vi "CSMP-Sync Call.vi"(0 "State":string, 1 "Args":string, 2 "Source/target":string, 5 "Error In":errorcluster caption="error in (no error)", 7 "Response Timeout (-2 Using Global Settings)":i32=-2, 8 "Module Name":string) -> (14 "State Out":string, 15 "Args Out":string, 16 "Source/target Out":string, 17 "Pre-State Out":string, 18 "Pre-Args Out":string, 19 "Error":errorcluster)   [LabVIEW 2017, in "Communicable State Machine.lvlib"]
doc: "### CSMP-Sync Call.vi\n\n-- <b>Controls</b> --\n- <b>state</b>:\n- <b>args</b>:\n- <b>source/target</b>:\n- <b>Response Timeout(-2 to use global setting)</b>:\n- <b>Module Name</b>:\n\n-- <b>Indicators</b> --\n- <b>state out</b>:\n- <b>args out</b>:\n- <b>source/target out</b>:\n- <b>Pre-State out</b>:\n- <b>Pre-Args out</b>:\n- <b>error</b>:"
uses:
  Communicable State Machine.lvlib
  Typedef/_Cross CSM State Data.ctl
  Typedef/_CSM_MSG_TYPE.ctl
  Typedef/_Cross CSM State Response.ctl
  Typedef/_CSM_Response Source Message.ctl
  _Shared/CSM - System States.vi
  Priority Queue/Enqueue Element.vi
  AdvanceAPI/CSM - Keywords.vi
  Error/CSM Not Allowed Message.vi
  CSMQ/_CSMOFGV(lvlibp).vi
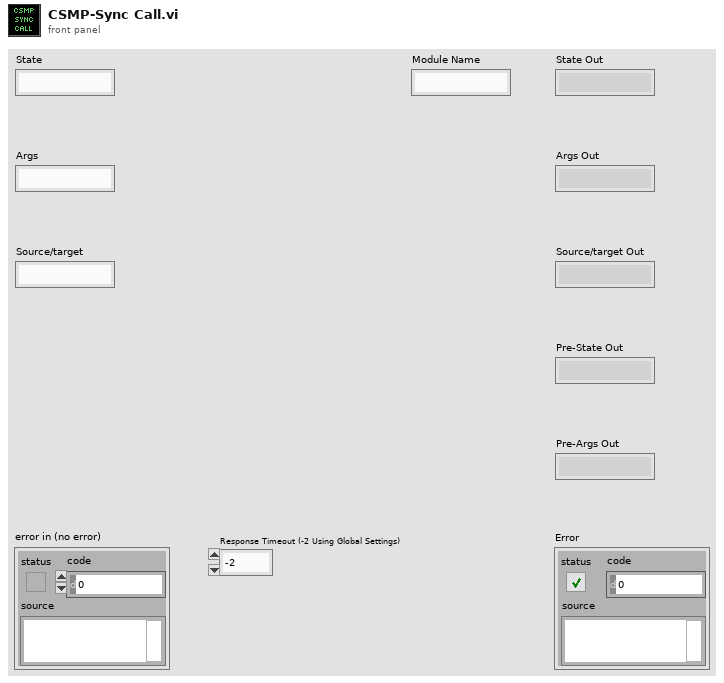
[diagram p1: front panel]
types:
  T1 = typedef "Communicable State Machine.lvlib/_CSMObj.ctl" = cluster{"info":T2, "Refs":T4}
  T2 = typedef "Communicable State Machine.lvlib/_CSMObj-Info.ctl" = cluster{"Module Name":string, "Requested Name":string, "Group Name":string, "Mode":T3, "Allowed Messages":string[]}
  T3 = typedef "Communicable State Machine.lvlib/_CSM_MODE.ctl" = enum16{"Not Exist", "Stand Alone", "CSM", "Worker", "Worker Agent", "Chain Node", "Chain"}
  T4 = typedef "Communicable State Machine.lvlib/_CSMObj-Refs.ctl" = cluster{"WatchDogQ":refnum<queue>, "CSMDataDVR":refnum<data-value>, "Queue":T5, "GroupDataDVR":refnum<data-value>, "TagMap":refnum<data-value>, "ExitEvent":refnum<user-event>, "NewStateEvent":refnum<user-event>, "StatusEvent":refnum<user-event>, "InterruptEvent":refnum<user-event>}
  T5 = typedef "Communicable State Machine.lvlib/Priority Queue.ctl" = cluster{"HPriorityQ":refnum<queue>, "LowPriorityQ":refnum<queue>}
  T6 = typedef "Communicable State Machine.lvlib/_Cross CSM State Response.ctl" = cluster{"error":errorcluster, "Response Data":string, "From Who":string}
  T7 = typedef "Communicable State Machine.lvlib/_CSM_MSG_TYPE.ctl" = enum16{"Sync Message(-@)", "Async Message(->)", "Async without Response(->|)", "Async Response", "Broadcast(-><all>)", "Broadcast(-><status>)", "Broadcast(-><interrupt>)", "Append to JKISM States", "Append to JKISM States(High Priority)", "Broadcast(-><state>)"}
  T8 = typedef "Communicable State Machine.lvlib/_Cross CSM State Data.ctl" = cluster{"Msg Type":T7, "state":string, "args":string, "source":string, "RespQ":refnum<queue>, "Response For Message":T9, "Target":string}
  T9 = typedef "Communicable State Machine.lvlib/_CSM_Response Source Message.ctl" = cluster{"‘State":string, "’Arguments":string, "’Error":errorcluster}
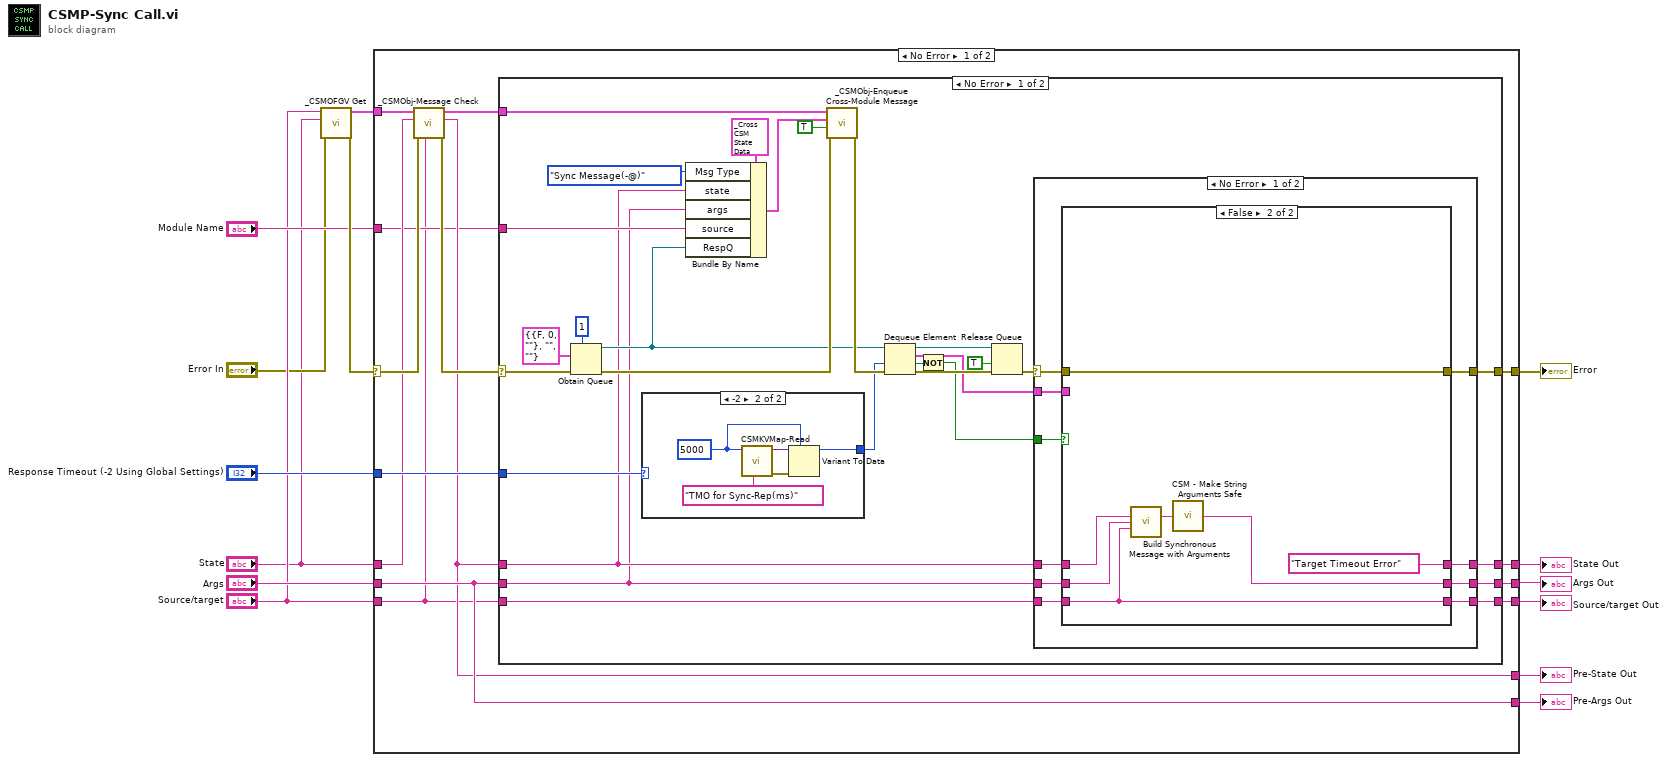
[diagram p0: block diagram]
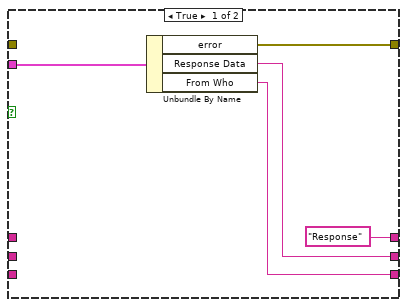
[diagram p2: hidden frame]
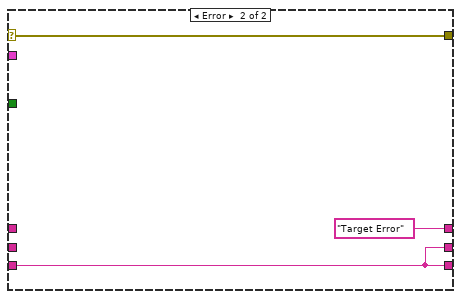
[diagram p3: hidden frame]
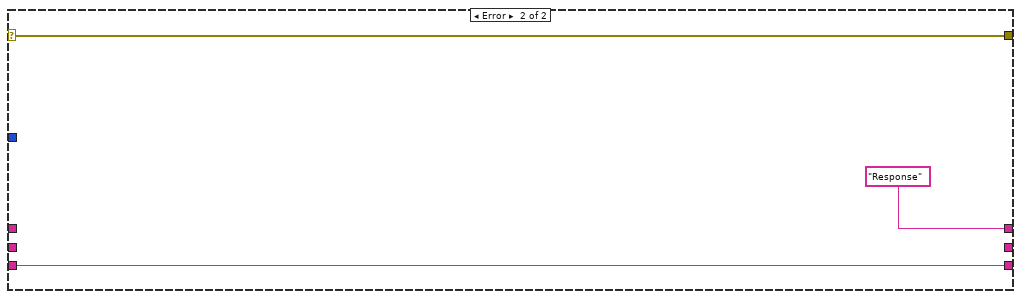
[diagram p5: hidden frame]
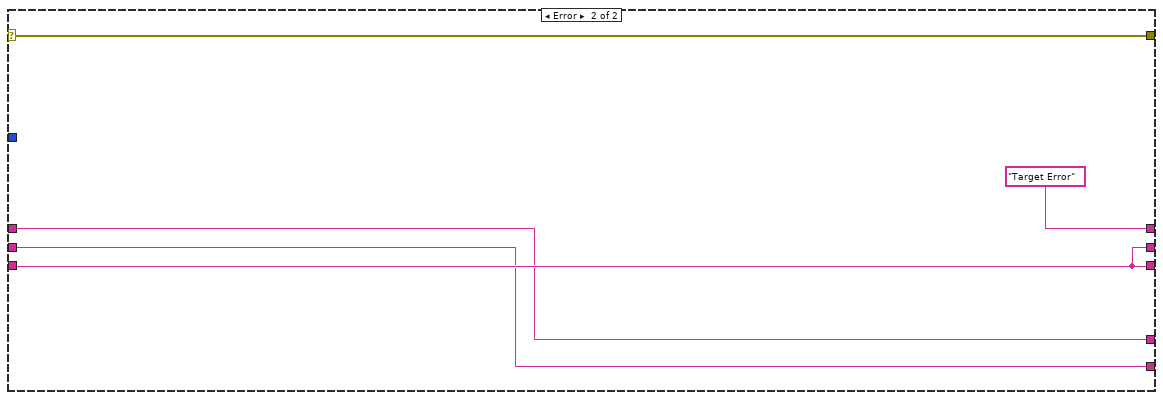
[diagram p6: hidden frame]
diagram:
  n1 = call "_CSMOFGV Get.vi"("Error In"="Error In", "Message"="State", "Name (\"\" to Use UUID) In"="Source/target") -> ("error out"=w13:errorcluster, "CSM-Obj"=w14:T1)  [unwired: 6 in, 1 out]
  n2 = case shown="No Error" w13 {
    selector: w13 -> [w20 w94]
    tunnel: "Response Timeout (-2 Using Global Settings)" -> [w28 _]
    tunnel: w14 -> [w22 _]
    tunnel: [w27 "Target Error" ("before match")] -> w8
    tunnel: [w26 w93] -> w7
    tunnel: "Source/target" -> [w15 w93]
    tunnel: "State" -> [w18 w92]
    tunnel: "Args" -> [w23 w91]
    tunnel: "Module Name" -> [w16 _]
    tunnel: [w23 w91] -> w5
    tunnel: [w25 w94] -> w4
    tunnel: [w17 w92] -> w6
    tunnel: [w24 w93] -> w2
    frame No Error {
      n3 = call "_CSMObj-Message Check.vi"("CSM"=w15, "Error In"=w20, "Message"=w18, "CSMQ In"=w22) -> ("error out"=w19:errorcluster, "Message (Dup)"=w17:string, "CSMQ Out"=w21:T1)  [unwired: 5 in]
      n4 = case shown="No Error" w19 {
        selector: w19 -> [w34 w90]
        tunnel: w28 -> [w32 _]
        tunnel: [w56 "Response" ("f")] -> w27
        tunnel: [w46 _] -> w26
        tunnel: w16 -> [w43 _]
        tunnel: w15 -> [w42 w88]
        tunnel: [w38 w90] -> w25
        tunnel: [w37 w88] -> w24
        tunnel: w23 -> [w29 _]
        tunnel: w21 -> [w35 _]
        tunnel: w17 -> [w30 _]
        frame No Error {
          n5 = Obtain Queue(max queue size (-1, unlimited)=1, element data type=T6 {"error"={"status"=FALSE, "code"=0, "source"=""}, "Response Data"="", "From Who"=""} ("Cross JKI State Machine Response"), error in (no error)=w34) -> (queue out=w45:refnum<queue>, error out=w48:errorcluster)  [unwired: 2 in, 1 out]
          n6 = case shown="-2" w32 {
            selector: w32 -> [w82 _]
            tunnel: [w82 w83] -> w31
            frame 0, Default {
            }
            frame -2 {
              w84 = 5000 ("max queue size (-1, unlimited)")
              n7 = call "CSMKVMap-Read.vi"("name"="TMO for Sync-Rep(ms)", "default value (empty variant)"=w84) -> ("Error out"=w87:errorcluster, "value"=w86:variant)  [unwired: 6 in]
              n8 = Variant To Data(error in=w87, type=w84, Variant=w86) -> (data=w83:i32)  [unwired: 1 out]
            }
          }
          n9 = Bundle By Name(cluster=T8 {"Msg Type"=enum."Sync Message(-@)", "state"="", "args"="", "source"="", "RespQ"=refnum, "Response For Message"={"‘State"="", "’Arguments"="", "’Error"={"status"=FALSE, "code"=0, "source"=""}}, "Target"=""} ("Cross JKI State Machine State"), "Msg Type"=_CSM_MSG_TYPE."Sync Message(-@)", "state"=w30, "args"=w29, "source"=w43, "RespQ"=w45) -> (w52:T8)
          n10 = call "_CSMObj-Enqueue Cross-Module Message.vi"("Error In"=w48, "High Priority? (F)"=TRUE ("High Priority?(F)"), "Data"=w52, "CSMQ In"=w35) -> ("error out"=w49:errorcluster)  [unwired: 6 in, 1 out]
          n11 = Dequeue Element(queue=w45, timeout in ms (-1)=w31, error in (no error)=w49) -> (queue out=w51:refnum<queue>, element=w47:T6, timed out?=w55:bool, error out=w50:errorcluster)
          n12 = Not(x=w55) -> (.not. x?=w41:bool)
          n13 = Release Queue(queue=w51, force destroy? (F)=TRUE, error in (no error)=w50) -> (error out=w36:errorcluster)  [unwired: 2 out]
          n14 = case shown="No Error" w36 {
            selector: w36 -> [w59 w80]
            tunnel: [w66 "Target Error" ("f")] -> w56
            tunnel: w47 -> [w65 _]
            tunnel: [w64 w79] -> w46
            tunnel: w42 -> [w63 w79]
            tunnel: w41 -> [w62 _]
            tunnel: [w61 w80] -> w38
            tunnel: [w60 w79] -> w37
            tunnel: w30 -> [w57 _]
            tunnel: w29 -> [w58 _]
            frame No Error {
              n15 = case shown="False" w62 {
                tunnel: ["Response" ("f") "Target Timeout Error" ("before match")] -> w66
                tunnel: w65 -> [w71 _]
                tunnel: [w68 w72] -> w64
                tunnel: w63 -> [_ w74]
                tunnel: [w70 w77] -> w61
                tunnel: [w67 w74] -> w60
                tunnel: w59 -> [_ w77]
                tunnel: w58 -> [_ w75]
                tunnel: w57 -> [_ w76]
                frame True {
                  n16 = Unbundle By Name(w71) -> ("error"=w70:errorcluster, "Response Data"=w68:string, "From Who"=w67:string)
                }
                frame False {
                  n17 = call "Build Synchronous Message with Arguments.vi"("State With Arguments"=w76, "Arguments (\"\")"=w75, "Target Module (\"\")"=w74) -> ("CSM Message String"=w73:string)  [unwired: 12 in]
                  n18 = call "CSM - Make String Arguments Safe.vi"("Argument String"=w73) -> ("Safe Argument String"=w72:string)  [unwired: 8 in]
                }
              }
            }
            frame Error {
            }
          }
        }
        frame Error {
        }
      }
    }
    frame Error {
    }
  }
  "State Out" <- w8
  "Args Out" <- w7
  "Source/target Out" <- w2
  "Pre-State Out" <- w6
  "Pre-Args Out" <- w5
  "Error" <- w4
